vi "Init.vi"(8 "error in (no error)":errorcluster, 11 "Socket":refnum<k5>) -> (0 "error out":errorcluster, 3 "Response out":refnum<class "Response.lvclass">)   [LabVIEW 2023, in "Response.lvclass"]
doc: "Creates an object that represents and manages the Response to an HTTP Request."
uses:
  Response.lvclass
  Response.lvclass/Response.ctl
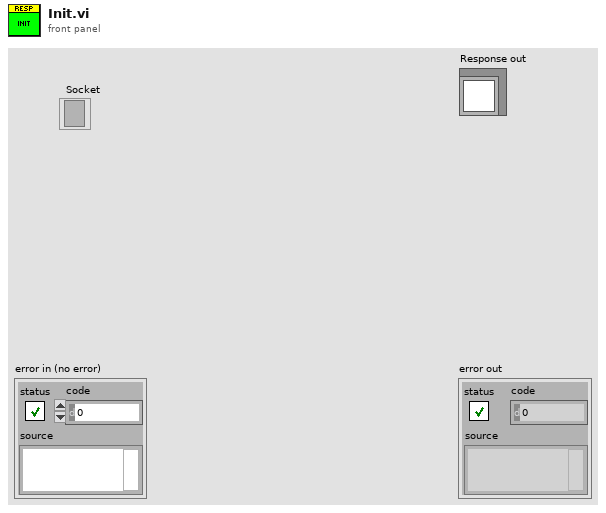
[diagram p1: front panel]
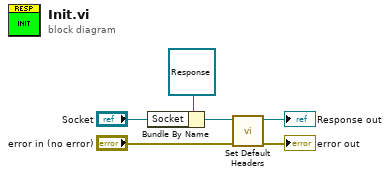
[diagram p0: block diagram]
diagram:
  n1 = Bundle By Name(cluster=refnum<class "Response.lvclass"> refnum ("Response in"), "Socket"="Socket") -> (w4:refnum<class "Response.lvclass">)
  n2 = call "Set Default Headers.vi"("error in (no error)"="error in (no error)", "Response in"=w4) -> ("error out"=→"error out":errorcluster, "Response out"=→"Response out":refnum<class "Response.lvclass">)  [unwired: 8 in]
